vi "Append Digital Trigger Name.vi"(8 "error in":errorcluster, 10 "Channels In":string[](array[string]), 11 "AnalogInput in":refnum<class "AnalogInput.lvclass">) -> (0 "error out":errorcluster, 2 "Channels Out":string[](array[string]), 3 "AnalogInput out":refnum<class "AnalogInput.lvclass">)   [LabVIEW 2019, in "AnalogInput.lvlib" / "AnalogInput.lvclass"]
uses:
  Library/AnalogInput.lvclass
  Library/AnalogInput.lvclass/AnalogInput.ctl
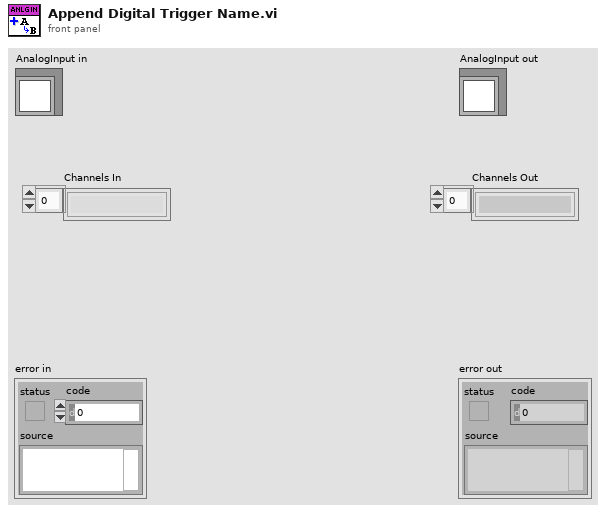
[diagram p1: front panel]
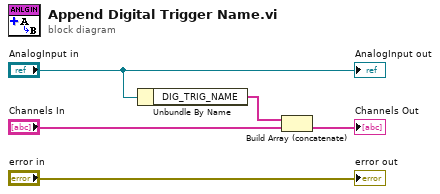
[diagram p0: block diagram]
diagram:
  n1 = Unbundle By Name("AnalogInput in") -> ("DIG_TRIG_NAME"=w1:string[])
  n2 = Build Array (concatenate)(w1, "Channels In") -> (→"Channels Out":string[])
  "error out" <- "error in"
  "AnalogInput out" <- "AnalogInput in"
